vi "CheckAndGetFIFOData.vi"(0 "DLL Path In":path, 1 "DataArryIn":u16[](array[numeric]), 5 "Module No. In":i16, 7 "Required No\nof Events":i32=2500, 9 "NoOfReadEventsIn":i32, 11 "Error In":errorcluster) -> (3 "DataArrayOut":u16[](array[numeric]), 4 "DLL Path Out":path, 6 "Module No. Out":i16, 8 "Busy":bool, 10 "NoOfReadEventsOut":i32, 13 "Col.TimerExpired":bool, 14 "Photon Count reached":bool, 15 "Error Out":errorcluster)   [LabVIEW 2023]
doc: "This convenience VIs wraps CheckState.vi and SPC_read_fifo.vi in one VI to provide a clearer code.\n<b>Attention: </b>this VI runs Inline to avoid memory allocation of SubVi calls.\n\ninfo@becker-hickl.com"
uses:
  SPC_Wrappers/Initialisation/SPC_get_error_string.vi
panel:
  # "Attention: this VI runs Inline to avoid memory allocation of SubVi calls"
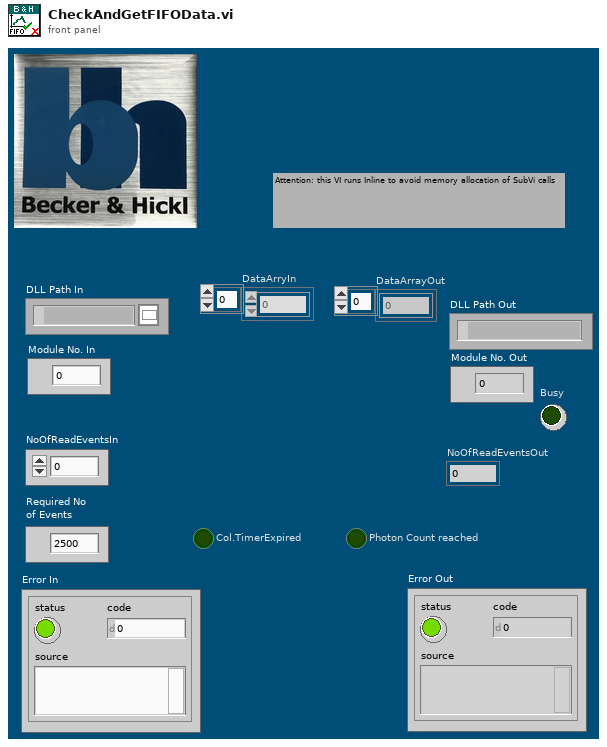
[diagram p1: front panel]
types:
  T1 = typedef "StateCluster.ctl" = cluster{"OVERFL":bool, "OVERFLOW":bool, "TIME_OVER":bool, "COLTIM_OVER":bool, "CMD_STOP":bool, "ARMED":bool, "REPTIM_OVER":bool, "COLTIM_2OVER":bool, "REPTIM_2OVER":bool, "FOVFL":bool, "FEMPTY":bool, "FBRDY":bool, "SCRDY":bool, "MEASURE":bool, "WAIT_TRG":bool, "HFILL_NRDY":bool, "SEQ_STOP":bool, "SEQ_GAP150":bool, "WAIT_FR":bool}
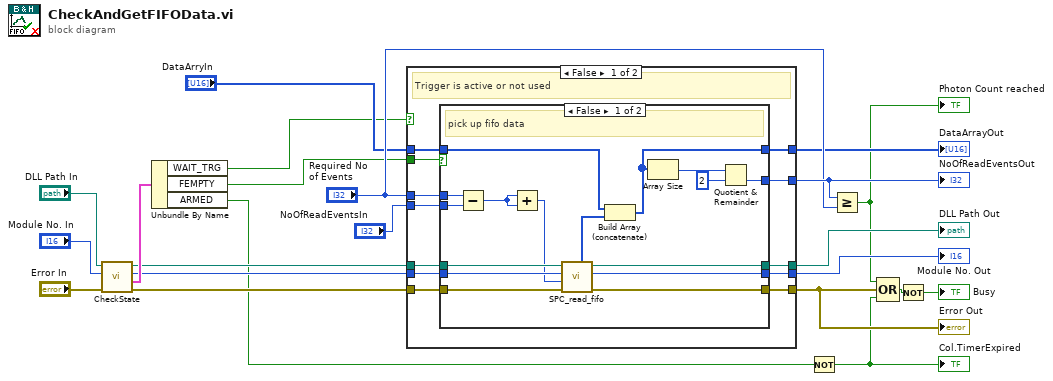
[diagram p0: block diagram]
diagram:
  n1 = call "CheckState.vi"("Error In"="Error In", "Module No."="Module No. In", "DLL Path"="DLL Path In") -> ("Error Out"=w17:errorcluster, "SPC_StateCluster"=w18:T1, "Module No."=w16:i16, "DLL Path"=w15:path)  [unwired: 4 in, 1 out]
  n2 = Unbundle By Name(w18) -> ("WAIT_TRG"=w4:bool, "FEMPTY"=w5:bool, "ARMED"=w2:bool)
  n3 = case shown="False" w4 {
    tunnel: w16 -> [w34 w56]
    tunnel: w17 -> [w33 w60]
    tunnel: [w32 w60] -> w6
    tunnel: [w31 w58] -> w7
    tunnel: [w30 w59] -> w20
    tunnel: "Required No\nof Events" -> [w29 _]
    tunnel: w15 -> [w28 w57]
    tunnel: w5 -> [w23 _]
    tunnel: "DataArryIn" -> [w27 w58]
    tunnel: "NoOfReadEventsIn" -> [w26 w59]
    tunnel: [w25 w57] -> w9
    tunnel: [w24 w56] -> w8
    frame False {
      # "Trigger is active or not used"
      n4 = case shown="False" w23 {
        tunnel: w34 -> [w50 w51]
        tunnel: w33 -> [w49 w55]
        tunnel: [w48 w55] -> w32
        tunnel: [w47 w54] -> w31
        tunnel: [w37 w53] -> w30
        tunnel: w29 -> [w46 _]
        tunnel: w28 -> [w45 w52]
        tunnel: w27 -> [w41 w54]
        tunnel: w26 -> [w40 w53]
        tunnel: [w43 w52] -> w25
        tunnel: [w42 w51] -> w24
        frame False {
          # "pick up fifo data"
          n5 = Subtract(x=w46, y=w40) -> (x-y=w35:i32)
          n6 = Add(x=w35, y=w35) -> (x+y=w36:i32)
          n7 = call "SPC_read_fifo.vi"("Error In"=w49, "Input Count"=w36, "Module No"=w50, "DLL Path"=w45) -> ("Error Out"=w48:errorcluster, "Module No"=w42:i16, "DLL Path"=w43:path, "Data Buffer"=w44:u16[])  [unwired: 3 in, 1 out]
          n8 = Build Array (concatenate)(w41, w44) -> (w47:u16[])
          n9 = Array Size(array=w47) -> (size(s)=w39:i32)
          n10 = Quotient & Remainder(x=w39, y=2) -> (floor(x/y)=w37:i32)  [unwired: 1 out]
        }
        frame True {
          # "Nothing to read"
        }
      }
    }
    frame True {
      # "Wait for trigger"
    }
  }
  "Error Out" <- w6
  "NoOfReadEventsOut" <- w20
  "DLL Path Out" <- w9
  "Module No. Out" <- w8
  "DataArrayOut" <- w7
  n11 = Not(x=w2) -> (.not. x?=w1:bool)
  "Col.TimerExpired" <- w1
  n12 = Greater Or Equal?(x=w20, y="Required No\nof Events") -> (x >= y?=w3:bool)
  "Photon Count reached" <- w3
  n13 = Compound Arithmetic op=OR(w3, w6, w1) -> (w22:bool)
  n14 = Not(x=w22) -> (.not. x?=→"Busy":bool)
